vi "Get Hardware Channels.vi"(8 "Error In":errorcluster, 10 "Index":u32, 11 "YAML Handle In":u64) -> (0 "Error Out":errorcluster, 2 "Hardware Channels":string, 3 "YAML Handle Out":u64)   [LabVIEW 2019, in "YAML Config Reader.lvlib"]
uses:
  YAML Config Reader.lvlib
  target/debug/rust_labview_yaml.dll
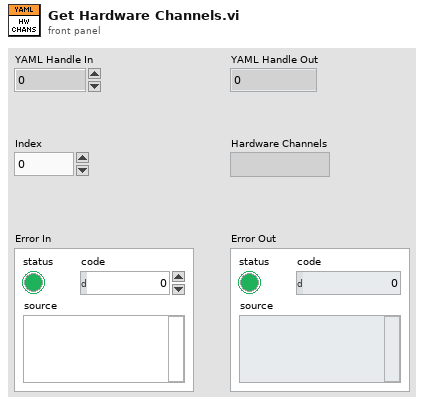
[diagram p1: front panel]
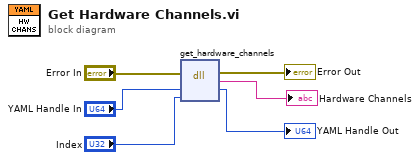
[diagram p0: block diagram]
diagram:
  n1 = dll-call lib="C:/dev/rust_labview_yaml/target/debug/rust_labview_yaml.dll" fn="get_hardware_channels"(error in="Error In", "DaqConfigurations"="YAML Handle In", "Index"="Index") -> (error out=→"Error Out":errorcluster, "Hardware Channels"=→"Hardware Channels":string, "DaqConfigurations"=→"YAML Handle Out":u64)  [unwired: 3 in, 1 out]
